vi "Create_Trajectory_Field_Crop_and_Scale.vi"(4 "Field Y Ft":dbl=27.0 format="%#_13g", 5 "Disp Y Size Pixel":i32=580, 6 "Field X Ft":dbl=54.0 format="%#_13g", 7 "Disp X Size Pixel":i32=1160, 9 "Field Image":T1, 10 "field Info":T2, 11 "Display Image":T1) -> (1 "Cropped Field Picture Out":picture, 2 "Full FIeld Image Out":T1, 3 "Filled Field Image Out":T1)   [LabVIEW 2020]
uses:
  TrajectoryUtils_Field_Info.ctl
  <vilib>/vision/Image Controls.llb/IMAQ Image.ctl
  <vilib>/vision/NI_Vision_Development_Module.lvlib
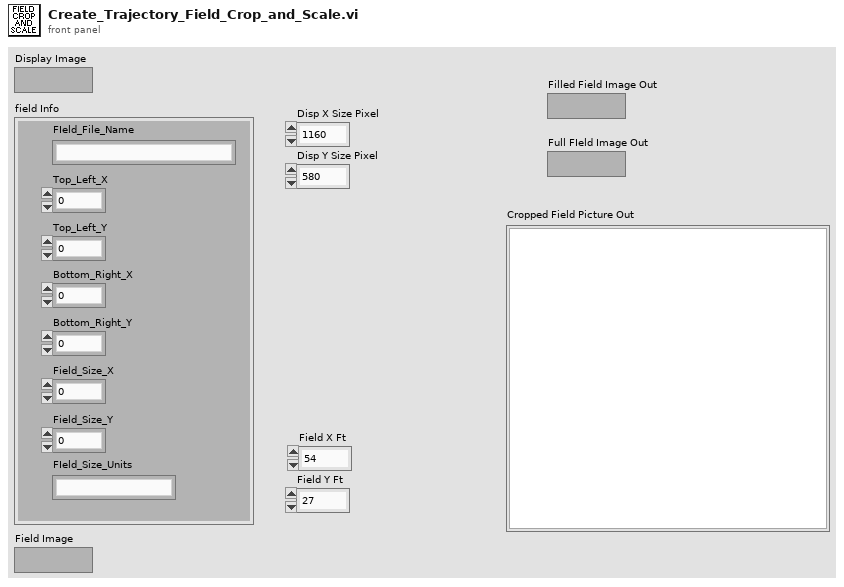
[diagram p1: front panel]
types:
  T1 = typedef "IMAQ Image.ctl" = refnum<image>
  T2 = typedef "TrajectoryUtils_Field_Info.ctl" = cluster{"FIeld_File_Name":string, "Top_Left_X":i32, "Top_Left_Y":i32, "Bottom_Right_X":i32, "Bottom_Right_Y":i32, "Field_Size_X":dbl, "Field_Size_Y":dbl, "FIeld_Size_Units":string}
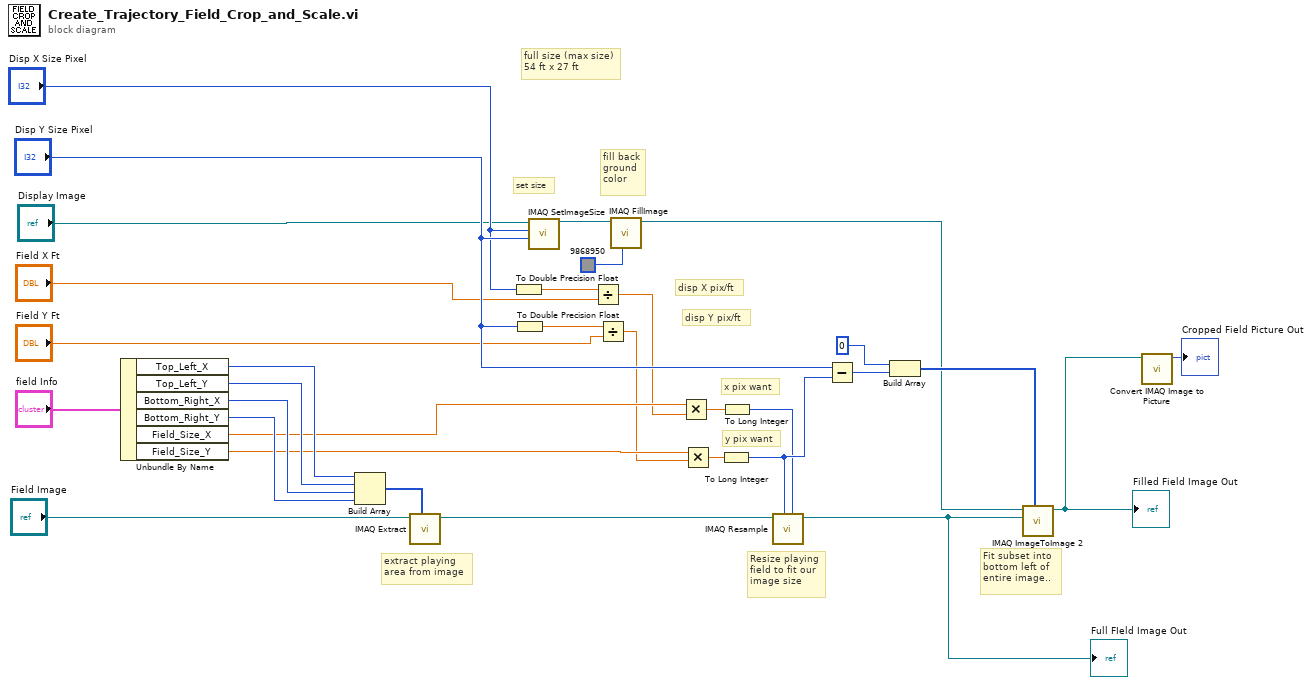
[diagram p0: block diagram]
diagram:
  # "Resize playing\nfield to fit our\nimage size"
  # "disp Y pix/ft"
  # "extract playing \narea from image"
  # "y pix want"
  # "x pix want"
  # "disp X pix/ft"
  # "fill back\nground\ncolor"
  # "set size"
  # "Fit subset into\nbottom left of \nentire image.."
  # "full size (max size)\n54 ft x 27 ft"
  n1 = Unbundle By Name("field Info") -> ("Top_Left_X"=w29:i32, "Top_Left_Y"=w30:i32, "Bottom_Right_X"=w31:i32, "Bottom_Right_Y"=w32:i32, "Field_Size_X"=w25:dbl, "Field_Size_Y"=w26:dbl)
  n2 = Build Array(w29, w30, w31, w32) -> (w4:i32[])
  n3 = call "IMAQ Extract"("Optional Rectangle"=w4, "Image Src"="Field Image") -> ("Image Dst Out"=w15:T1)  [unwired: 8 in, 1 out]
  n4 = To Double Precision Float(number="Disp X Size Pixel") -> (double precision float=w9:dbl)
  n5 = To Double Precision Float(number="Disp Y Size Pixel") -> (double precision float=w10:dbl)
  n6 = call "IMAQ SetImageSize"("Y Resolution"="Disp Y Size Pixel", "X Resolution"="Disp X Size Pixel", "Image"="Display Image") -> ("Image Out"=w6:T1)  [unwired: 2 in, 1 out]
  n7 = Divide(x=w9, y="Field X Ft") -> (x/y=w13:dbl)
  n8 = Divide(x=w10, y="Field Y Ft") -> (x/y=w14:dbl)
  n9 = call "IMAQ FillImage"("Color Pixel Value"=u32 9868950, "Image"=w6) -> ("Image Out"=w19:T1)  [unwired: 8 in, 1 out]
  n10 = Multiply(x=w25, y=w13) -> (x*y=w17:dbl)
  n11 = Multiply(x=w26, y=w14) -> (x*y=w18:dbl)
  n12 = To Long Integer(number=w18) -> (32bit integer=w22:i32)
  n13 = To Long Integer(number=w17) -> (32bit integer=w16:i32)
  n14 = call "IMAQ Resample"("X Resolution"=w16, "Y Resolution"=w22, "Image Src"=w15) -> ("Image Dst Out"=w23:T1)  [unwired: 7 in, 1 out]
  "Full FIeld Image Out" <- w23
  n15 = Subtract(x="Disp Y Size Pixel", y=w22) -> (x-y=w27:i32)
  n16 = Build Array(0, w27) -> (w24:i32[])
  n17 = call "IMAQ ImageToImage 2"("Offset Left/Top"=w24, "Image Src (Small)"=w23, "Image Src (Large)"=w19) -> ("Image Dst Out"=w2:T1)  [unwired: 7 in, 1 out]
  "Filled Field Image Out" <- w2
  n18 = call "Convert IMAQ Image to Picture.vi"("Image In"=w2) -> ("new picture"=→"Cropped Field Picture Out":picture)  [unwired: 10 in]
